vi "Control Events.vi"(8 "error in (no error)":errorcluster, 11 "Control in":refnum<class "Control.lvclass">) -> (0 "error out":errorcluster, 2 "Control Events":refnum<class "Control Event Registrations.lvclass">, 3 "Control out":refnum<class "Control.lvclass">)   [LabVIEW 2020, in "VolatusGUI.lvlib" / "Control.lvclass"]
uses:
  Control.lvclass
  Control.lvclass/Control.ctl
  Control Event Registrations/Control Event Registrations.lvclass
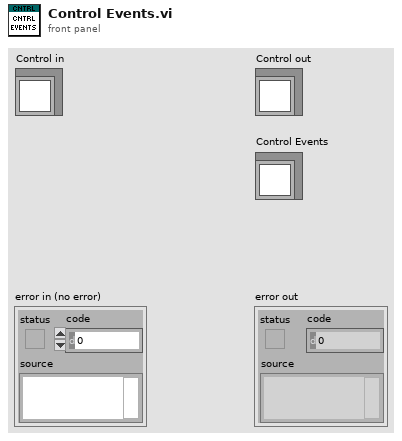
[diagram p1: front panel]
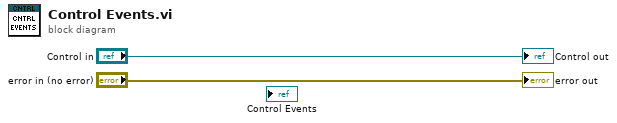
[diagram p0: block diagram]
diagram:
  "error out" <- "error in (no error)"
  "Control out" <- "Control in"
